vi "ConvertTextBasedCodeToLabVIEW_RemoveUnitTestTags.vi"(11 "TextIn":string) -> (3 "TextOut":string)   [LabVIEW 2020]
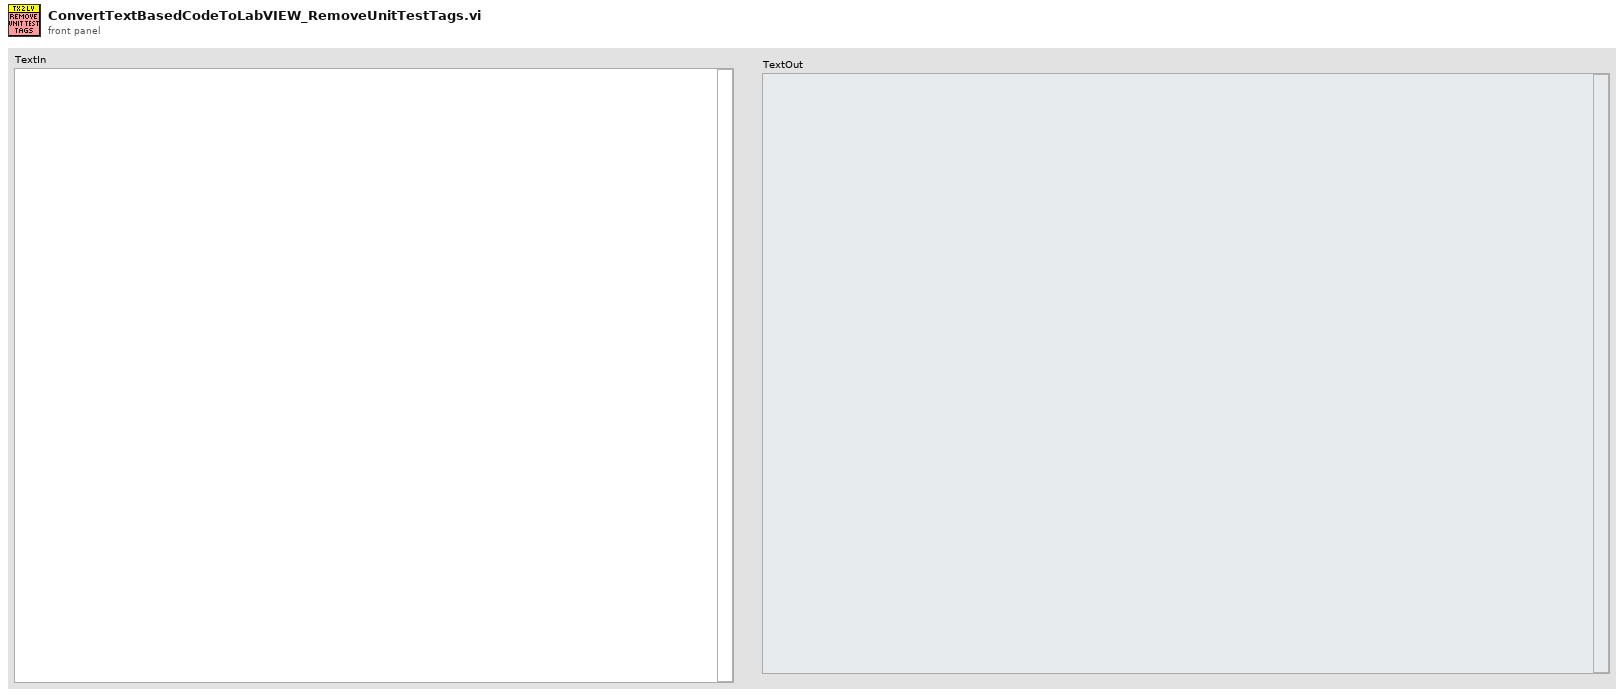
[diagram p1: front panel]
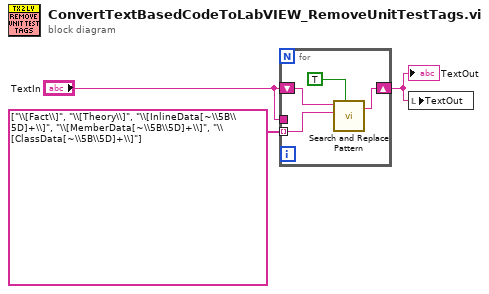
[diagram p0: block diagram]
diagram:
  n1 = for {
    tunnel: string[] ["\\[Fact\\]", "\\[Theory\\]", "\\[InlineData[~\\5B\\5D]+\\]", "\\[MemberData[~\\5B\\5D]+\\]", "\\[ClassData[~\\5B\\5D]+\\]"] ("input string") -> [w4] mode=indexing
    tunnel: "TextIn" -> [_]
    shift-right: [w6] -> w1
    shift-left: "TextIn" -> [w7]
    n2 = call <vilib>:"Search and Replace Pattern.vi"("string"=w7, "regular expression (\"\")"=w4, "replace all? (F)"=TRUE) -> ("result string"=w6:string)  [unwired: 2 in, 1 out]
  }
  "TextOut" <- w1
  n3 = local write "TextOut"(w1) -> ()
